vi "Continuous Serial Write and Read Yohav.vi"() -> ()   [LabVIEW 2017]
doc: "This example performs writes and reads on a serial port, as directed by the user. You can press the Write and Read buttons, and change the Read Count, while the example is running.\n\nThe parameters set for the serial port must match the parameters of the connected instrument or device. In this example, the Read Count parameter specifies the number of bytes that the serial port reads. If there were more bytes at the port than the specified number, those bytes would not be read. If there were less bytes at the port than the specified number, you would receive a timeout error.\n\nThis example expands upon the flow control options for XON and XOFF, allowing the user to choose those control characters. Also, the user can enable or disable a termination character. Some devices require a termination character in order to identify the end of command strings. Some devices send a termination character to signify the end of data to be read. This example shows how you can end the Read operation once a termination character is detected in the buffer and/or append a termination character at the end of the Write data."
uses:
  Program Files (x86)/National Instruments/LabVIEW 2017/examples/Instrument IO/Serial/support/Serial - Settings.ctl
  Program Files (x86)/National Instruments/LabVIEW 2017/examples/Instrument IO/Serial/support/Serial - XON-XOFF Characters.ctl
  Program Files (x86)/National Instruments/LabVIEW 2017/examples/Instrument IO/Serial/support/Serial - ASCII Characters.ctl
  <vilib>/Instr/_visa.llb/VISA Configure Serial Port (Instr).vi
panel:
  out "string":string
  in  "Byte #2":u8
  in  "Array":u8[](array[numeric]) format="%.0x"
  out "return count":u32
  in  "Clear":bool
  in  "Termination Character":u8=10 format="%.0x"
  in  "End Write on Termination Character?":bool=TRUE
  in  "Stop":bool
  in  "Command":string="*IDN?"
  in  "Read Count":u32=1000
  out "Response":string
  in  "Write":bool
  in  "Read":bool
  in  "XON/XOFF Characters":T1={"XON"=enum."DC1", "XOFF"=enum."DC3"}
  in  "Serial Settings":T3={"baud rate"=57600, "data bits"=8, "parity"=enum."None", "stop bits"=10, "flow control"=0} {"flow control" items=["None"=0, "XON/XOFF"=1, "RTS/CTS"=2, "DTR/DSR"=4]; "stop bits" items=["1.0"=10, "1.5"=15, "2.0"=20]; "data bits" min=5 max=8 step=1; "baud rate" items=["75"=75, "110"=110, "134"=134, "150"=150, "300"=300, "600"=600, "1200"=1200, "1800"=1800, "2400"=2400, "4800"=4800, "7200"=7200, "9600"=9600, "14400"=14400, "19200"=19200, "28800"=28800, "38400"=38400, "56000"=56000, "57600"=57600, "115200"=115200, "128000"=128000, "230400"=230400]}
  in  "End Read on Termination Character?":bool=TRUE
  in  "VISA resource name":refnum<visa-resource-name>="COM1"
  # "Overview: Demonstrates the use of the VISA functions to write commands to and read responses from a serial instrument continuously in a loop.\nRequirements: NI-VISA Driver\nInstructions:\n1. Run the VI.\n2. Specify a Command and click the Write button.\n3. Read a Response by clicking the Read button.\n4. Click Stop to stop the VI."
  # "0xA is equivalent to a '\\n' character, which is a line feed."
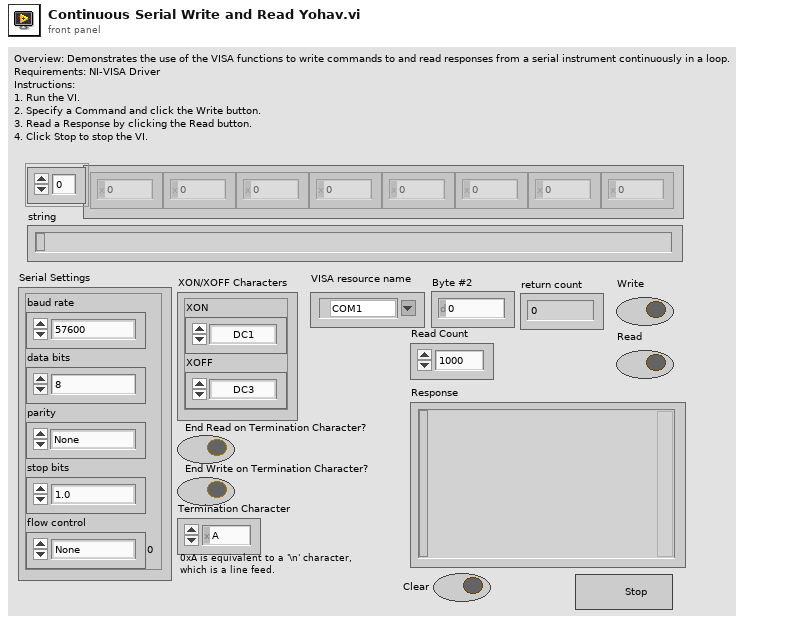
[diagram p1: front panel]
types:
  T1 = typedef "Serial - XON-XOFF Characters.ctl" = cluster{"XON":T2, "XOFF":T2}
  T2 = typedef "Serial - ASCII Characters.ctl" = enum16{"NUL", "SOH", "STX", "ETX", "EOT", "ENQ", "ACK", "BEL", "BS", "HT", "LF", "VT", "FF", "CR", "SO", "SI", "DLE", "DC1", "DC2", "DC3", "DC4", "NAK", "SYN", "ETB", "CAN", "EM", "SUB", "ESC", "FS", "GS", "RS", "US", "SP", "!", "\"", "#", "$", "%", "&", "'", "(", ")", "*", "+", ",", "- (-)", ".", "/", "0", "1", "2", "3", "4", "5", "6", "7", "8", "9", ":", ";", "<", "=", ">", "?", "@", "A", "B", "C", "D", "E", "F", "G", "H", "I", "J", "K", "L", "M", "N", "O", "P", "Q", "R", "S", "T", "U", "V", "W", "X", "Y", "Z", "[", "\\", "]", "^", "_", "`", "a", "b", "c", "d", "e", "f", "g", "h", "i", "j", "k", "l", "m", "n", "o", "p", "q", "r", "s", "t", "u", "v", "w", "x", "y", "z", "{", "|", "}", "~"}
  T3 = typedef "Serial - Settings.ctl" = cluster{"baud rate":u32, "data bits":u16, "parity":enum16{"None", "Odd", "Even", "Mark", "Space"}, "stop bits":u16, "flow control":u16}
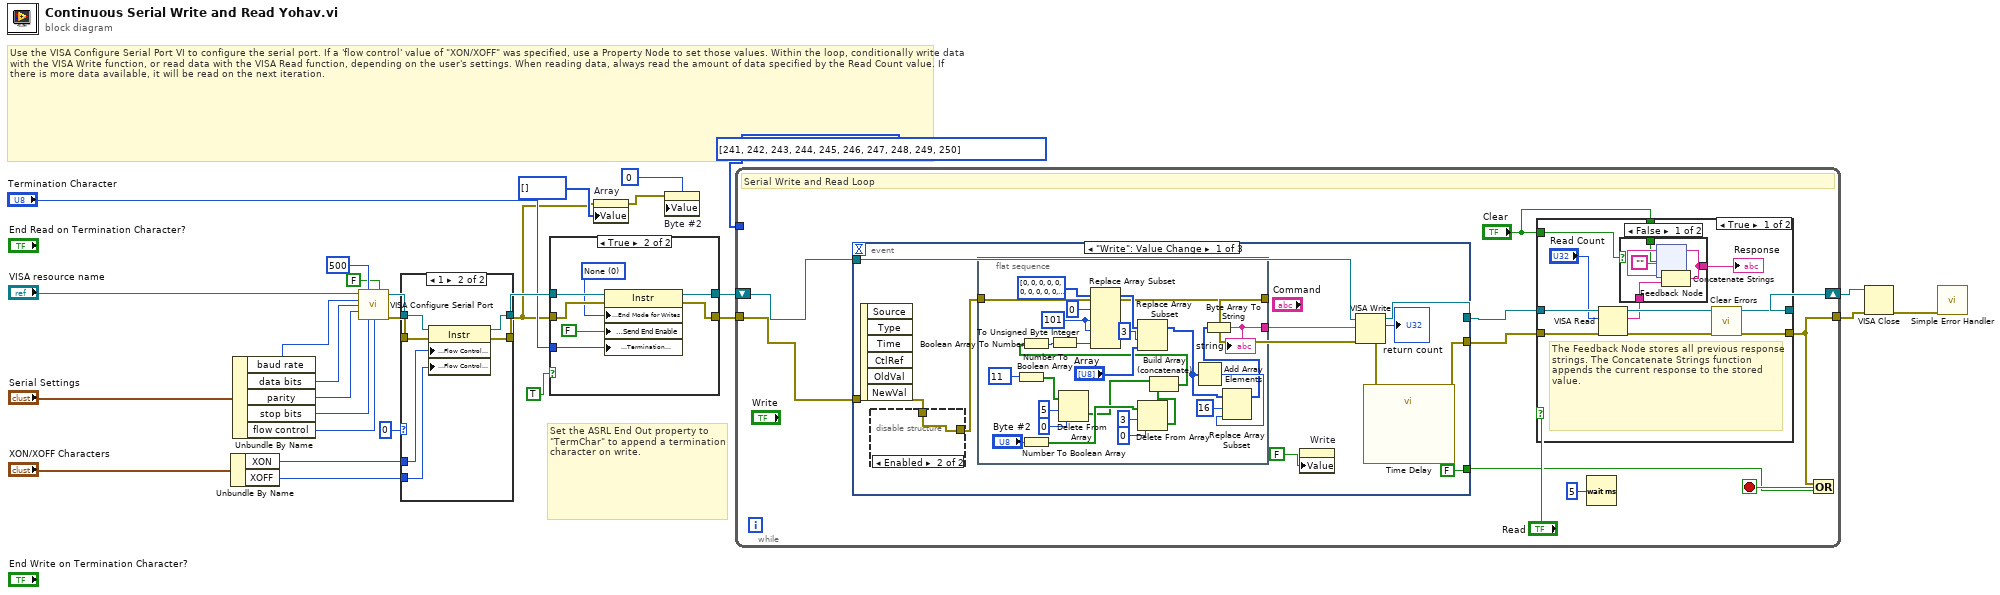
[diagram p0: block diagram]
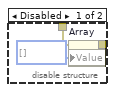
[diagram p4: hidden frame]
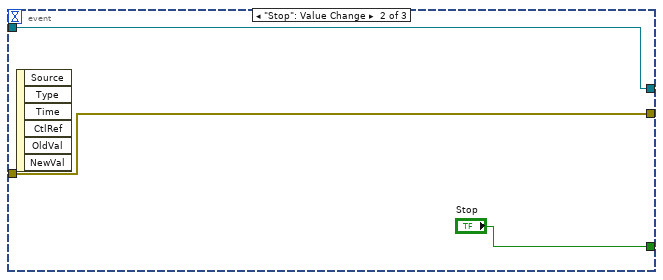
[diagram p5: hidden frame]
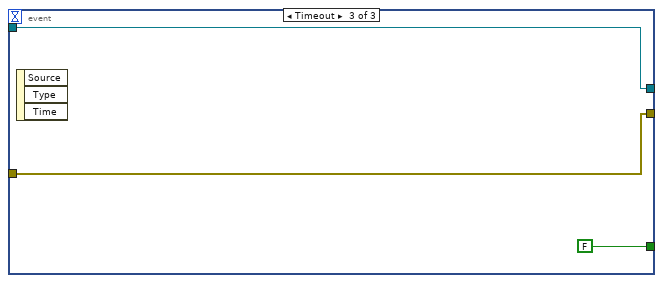
[diagram p6: hidden frame]
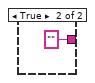
[diagram p7: hidden frame]
diagram:
  # "Set the ASRL End Out property to \"TermChar\" to append a termination character on write."
  # "Use the VISA Configure Serial Port VI to configure the serial port. If a 'flow control' value of \"XON/XOFF\" was specified, use a Property Node to set those values. Within the loop, conditionally write data with the VISA Write function, or read data with the VISA Read function, depending on the user's settings. When reading data, always read the amount of data specified by the Read Count value. If there is more data available, it will be read on the next iteration."
  n1 = Unbundle By Name("XON/XOFF Characters") -> ("XON"=w15:T2, "XOFF"=w14:T2)
  n2 = Unbundle By Name("Serial Settings") -> ("baud rate"=w21:u32, "data bits"=w22:u16, "parity"=w23:enum16{"None", "Odd", "Even", "Mark", "Space"}, "stop bits"=w24:u16, "flow control"=w16:u16)
  n3 = call-poly "VISA Configure Serial Port"("VISA resource name"="VISA resource name", "timeout (10sec)"=u32 500, "Enable Termination\nChar (T)"=FALSE ("Enable Termination\nChar (T)"), "baud rate (9600)"=w21, "data bits (8)"=w22, "parity (0:none)"=w23, "stop bits (10: 1 bit)"=w24, "flow control (0:none)"=w16) -> ("VISA resource name out"=w25:refnum<visa-resource-name>, "error out"=w26:errorcluster)  [unwired: 2 in, 4 out]
  n4 = case shown="1" u16 0 ("flow control") {
    tunnel: [w29 w36] -> w2
    tunnel: [w30 w35] -> w12
    tunnel: w26 -> [w29 w34]
    tunnel: w25 -> [w30 w33]
    tunnel: w15 -> [_ w32]
    tunnel: w14 -> [_ w31]
    frame Default {
    }
    frame 1 {
      n5 = property class="Instr"(reference=w33, error in=w34, "Serial Settings:Flow Control XON Character"=w32, "Serial Settings:Flow Control XOFF Character"=w31) -> (reference out=w35:refnum<visa-resource-name>, error out=w36:errorcluster)
    }
  }
  n6 = case shown="True" TRUE {
    tunnel: w12 -> [w37 w45]
    tunnel: w2 -> [w38 w44]
    tunnel: [w37 w43] -> w11
    tunnel: [w38 w42] -> w13
    tunnel: "Termination Character" -> [_ w40]
    frame False {
    }
    frame True {
      w41 = u16 0 items=["None", "LastBit", "TermChar", "Break"] ("Serial Settings:Serial End Mode for Writes")
      n7 = property class="Instr"(reference=w45, error in=w44, "Serial Settings:End Mode for Writes"=w41, "Message Based Settings:Send End Enable"=FALSE, "Message Based Settings:Termination Character"=w40) -> (reference out=w43:refnum<visa-resource-name>, error out=w42:errorcluster)
    }
  }
  n8 = property on="Array" class="Arr (strict)"(error in=w2, "Value"=u8[] []) -> (error out=w1:errorcluster)  [unwired: 1 in, 1 out]
  n9 = property on="Byte #2" class="DigNum (strict)"(error in=w1, "Value"=u8 0 ("Byte #2")) -> ()  [unwired: 1 in, 2 out]
  n10 = while {
    shift-right: [w56] -> w17
    shift-left: w11 -> [w55]
    tunnel: w13 -> [w54]
    tunnel: [w49] -> w18
    tunnel: u8[] [241, 242, 243, 244, 245, 246, 247, 248, 249, 250] -> [_]
    stop <- w50 stop-if-true
    # "Serial Write and Read Loop"
    n11 = event shown="[0] \"Write\": Value Change" {
      selector: _ -> [_ _ _]
      dyn-events: _ -> [_ _ _]
      timeout: _ -> [_ _ _]
      tunnel: w55 -> [w67 w98 w102]
      tunnel: w54 -> [w59 w97 w101]
      tunnel: [w66 w98 w102] -> w53
      tunnel: [w64 w97 w101] -> w46
      tunnel: [FALSE ("Stop") "Stop" FALSE ("Stop")] -> w47
      event "Write": Value Change {
        n12 = event-data() -> ()  [unwired: 1 in, 6 out]
        n13 = disable-structure shown="Enabled" {
          disable-tunnel: w59 -> [w69 w71]
          disable-tunnel: [w68 w71] -> w57
          frame Disabled {
            n14 = property on="Array" class="Arr (strict)"(error in=w69, "Value"=u8[] []) -> (error out=w68:errorcluster)  [unwired: 1 in, 1 out]
          }
          frame Enabled {
          }
        }
        n15 = flat-sequence {
          tunnel: [w96] -> w62
          tunnel: [w78] -> w58
          tunnel: w57 -> [w78]
          frame #0 {
            w77 = u8 101 ("new element/subarray")
            n16 = Number To Boolean Array(number=u8 11) -> (Boolean array=w87:bool[])
            n17 = Number To Boolean Array(number="Byte #2") -> (Boolean array=w82:bool[])
            n18 = Delete From Array(array=w87, length=5, index=0) -> (deleted portion=w81:bool[])  [unwired: 1 out]
            n19 = Delete From Array(array=w82, length=3, index=0) -> (deleted portion=w80:bool[])  [unwired: 1 out]
            n20 = Build Array (concatenate)(w81, w80) -> (w79:bool[])
            n21 = Boolean Array To Number(Boolean array=w79) -> (number=w94:u32)
            n22 = To Unsigned Byte Integer(number=w94) -> (unsigned 8bit integer=w76:u8)
            n23 = Replace Array Subset(array=u8[] [0, 0, 0, 0, 0, 0, 0, 0, 0, 0, 0, 0, 0, 0, 0, 0, 0], new element #1=w77, index #1=0 ("index"), new element #2=w77, new element #3=w76) -> (w90:u8[])  [unwired: 2 in]
            n24 = Replace Array Subset(array=w90, new element="Array", index=3) -> (w74:u8[])
            n25 = Add Array Elements(numeric array=w74) -> (sum=w73:u8)
            n26 = Replace Array Subset(array=w74, new element=w73, index=16) -> (w72:u8[])
            n27 = Byte Array To String(unsigned byte array=w72) -> (string=w96:string)
            "string" <- w96
          }
        }
        n28 = property on="Write" class="Bool (strict)"("Value"=FALSE ("Write")) -> ()  [unwired: 2 in, 2 out]
        n29 = VISA Write(VISA resource name=w67, write buffer=w62, error in (no error)=w58) -> (VISA resource name out=w66:refnum<visa-resource-name>, return count=→"return count":u32, error out=w65:errorcluster)
        n30 = call "Time Delay"("error in (no error)"=w65) -> ("error out"=w64:errorcluster)  [unwired: 10 in]
      }
      event "Stop": Value Change {
        n31 = event-data() -> ()  [unwired: 1 in, 6 out]
      }
      event Timeout {
        n32 = event-data() -> ()  [unwired: 1 in, 3 out]
      }
    }
    n33 = case shown="True" "Read" {
      tunnel: [w110 w120] -> w56
      tunnel: w53 -> [w112 w120]
      tunnel: [w105 w119] -> w49
      tunnel: w46 -> [w111 w119]
      tunnel: "Clear" -> [w104 _]
      tunnel: "Clear" -> [w103 _]
      frame True {
        # "The Feedback Node stores all previous response strings. The Concatenate Strings function appends the current response to the stored value."
        n34 = VISA Read(VISA resource name=w112, byte count="Read Count", error in (no error)=w111) -> (VISA resource name out=w110:refnum<visa-resource-name>, read buffer=w107:string, error out=w108:errorcluster)  [unwired: 1 out]
        n35 = case shown="False" w104 {
          tunnel: w107 -> [w117 _]
          tunnel: [w115 ""] -> w106
          tunnel: w103 -> [w113 _]
          frame False {
            n36 = feedback #1("") -> (w116:string)
            n37 = Concatenate Strings(w116, w117) -> (w115:string)
            n38 = feedback-in #1(w115, w113) -> ()
          }
          frame True {
          }
        }
        "Response" <- w106
        n39 = call <vilib>:"Clear Errors.vi"("error in (no error)"=w108) -> ("error out"=w105:errorcluster)  [unwired: 5 in, 1 out]
      }
      frame False {
      }
    }
    n40 = Wait (ms)(milliseconds to wait=u32 5) -> ()  [unwired: 1 out]
    n41 = Or(x=w49, y=w47) -> (x .or. y?=w50:bool)
  }
  n42 = VISA Close(VISA resource name=w17, error in (no error)=w18) -> (error out=w19:errorcluster)
  n43 = call <vilib>:"Simple Error Handler.vi"("error in (no error)"=w19) -> ()  [unwired: 1 in, 8 out]
